vi "Get uSs List in current Run Config.vi"(8 "error in (no error)":errorcluster, 11 "Guardian in":refnum<class "Guardian.lvclass">) -> (0 "error out":errorcluster, 2 "uSs in Run Config":string[](array[string]), 3 "Guardian out":refnum<class "Guardian.lvclass">)   [LabVIEW 2026, in "TALOS.lvlib" / "Guardian.lvlib" / "Guardian.lvclass"]
uses:
  Guardian.lvclass
  Guardian.lvclass/Guardian.ctl
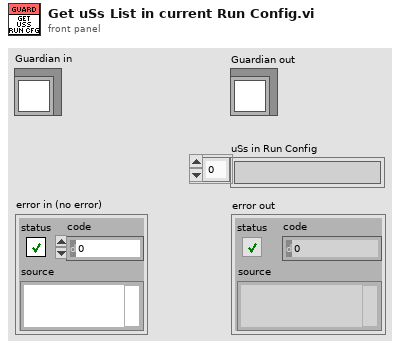
[diagram p1: front panel]
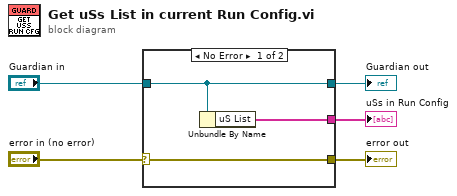
[diagram p0: block diagram]
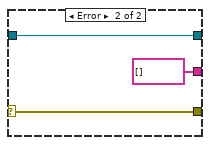
[diagram p2: hidden frame]
diagram:
  n1 = case shown="No Error" "error in (no error)" {
    selector: "error in (no error)" -> [w7 w9]
    tunnel: "Guardian in" -> [w6 w11]
    tunnel: [w6 w11] -> w3
    tunnel: [w7 w9] -> w2
    tunnel: [w8 string[] [] ("uS array")] -> w1
    frame No Error {
      n2 = Unbundle By Name(w6) -> ("uS List"=w8:string[])
    }
    frame Error {
    }
  }
  "Guardian out" <- w3
  "error out" <- w2
  "uSs in Run Config" <- w1
